vi "EventLogger.Error.vi"(7 "Flush To Disk On Error":bool, 8 "error in":errorcluster) -> (0 "error out":errorcluster)   [LabVIEW 2019, in "Tools.lvlib"]
uses:
  Tools.lvlib
  <vilib>/NI/Event Logger Library/EventLog/EventLog.lvclass
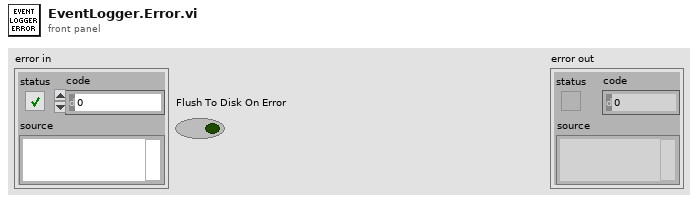
[diagram p1: front panel]
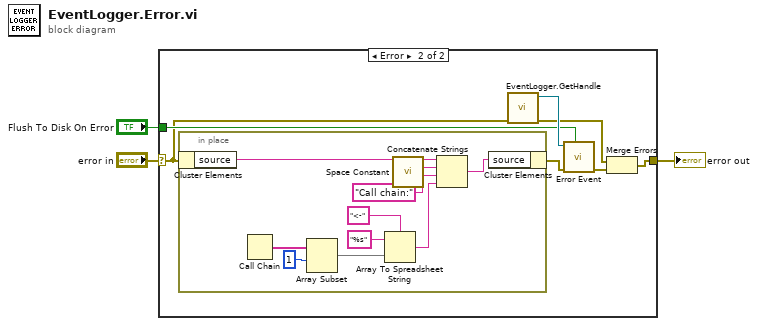
[diagram p0: block diagram]
diagram:
  n1 = case shown="Error" "error in" {
    selector: "error in" -> [w4 w5]
    tunnel: "Flush To Disk On Error" -> [_ w9]
    tunnel: [w4 w8] -> w2
    frame No Error {
    }
    frame Error {
      n2 = in-place {
        n3 = in-place-cluster #1(w5) -> ("source"=w21:string)
        n4 = Call Chain() -> (call chain=w17:string[])
        n5 = Array Subset(array=w17, index=1) -> (w14:string[])  [unwired: 1 in]
        n6 = Array To Spreadsheet String(delimiter (Tab)="<-", array=w14, 3:"%s" ("format string")) -> (spreadsheet string=w15:string)
        n7 = call <vilib>:"Space Constant.vi"() -> ("String"=w20:string)
        n8 = Concatenate Strings(w21, w20, "Call chain:" ("string"), w15) -> (w18:string)
        n9 = in-place-cluster #1("source"=w18) -> (w6:errorcluster)
      }
      n10 = call "EventLogger.GetHandle.vi"("error in"=w5) -> ("error out"=w7:errorcluster, "EventLog ref"=w11:refnum<class "EventLog.lvclass">)  [unwired: 9 in]
      n11 = call <vilib>:"Error Event.vi"("Flush To Disk On Error"=w9, "error in (no error)"=w6, "EventLog ref"=w11) -> ("error out"=w10:errorcluster)  [unwired: 7 in, 1 out]
      n12 = Merge Errors(w7, w10) -> (w8:errorcluster)
    }
  }
  "error out" <- w2
